vi "validate line configuration.vi"(7 "EthernetIP configuration":refnum<class "EthernetIP configuration.lvclass">, 11 "line in":T1) -> (1 "valid?":bool, 2 "problem":string, 3 "line out":T1)   [LabVIEW 2013, in "EthernetIP editor node.lvclass"]
uses:
  EthernetIP editor node.lvclass
  table line.ctl
  <vilib>/NI/TBM Modules/Ethernet IP/channel/EthernetIP Channel.lvclass
  <vilib>/NI/TBM Modules/Ethernet IP/configuration/EthernetIP configuration.lvclass
  <vilib>/NI/Tag Bus/tag/tag descriptor.lvclass/tag descriptor.ctl
  <vilib>/NI/TBM Modules/Ethernet IP/channel/EthernetIP Channel.lvclass/EthernetIP Channel.ctl
  <vilib>/NI/Tag Bus Module Framework/channel/TBM channel.lvclass/TBM channel.ctl
  <vilib>/NI/TBM Modules/Ethernet IP/configuration/EthernetIP configuration.lvclass/EthernetIP configuration.ctl
  <vilib>/NI/TBM Modules/Ethernet IP/configuration/read eip channels.vi
  <vilib>/NI/TBM Modules/Ethernet IP/configuration/Read assemblies.vi
  <vilib>/NI/Tag Bus/tag/read tag name.vi
  <vilib>/NI/TBM Modules/Ethernet IP/channel/Read Instance ID.vi
  <vilib>/NI/Tag Bus Module Framework/channel/Read channel classification.vi
  <vilib>/NI/TBM Modules/Ethernet IP/channel/Read subindex.vi
  <vilib>/NI/Tag Bus/tag/tag descriptor.lvclass
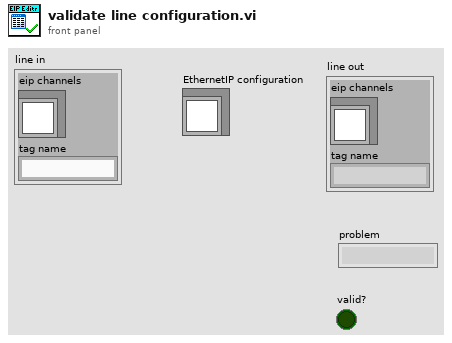
[diagram p1: front panel]
types:
  T1 = typedef "EthernetIP editor node.lvclass/table line.ctl" = cluster{"eip channels":refnum<class "EthernetIP Channel.lvclass">, "tag name":string}
  T2 = typedef "TBM channel.lvclass/channel classification.ctl" = enum16{"input data", "output data", "processing parameter", "processing result"}
  T3 = typedef "EthernetIP configuration.lvclass/assembly definition.ctl" = cluster{"name":string, "Instance ID":u32, "Type":T4, "Size (bytes)":u32}
  T4 = typedef "EthernetIP configuration.lvclass/assembly type.ctl" = enum32{"Producing", "Consuming"}
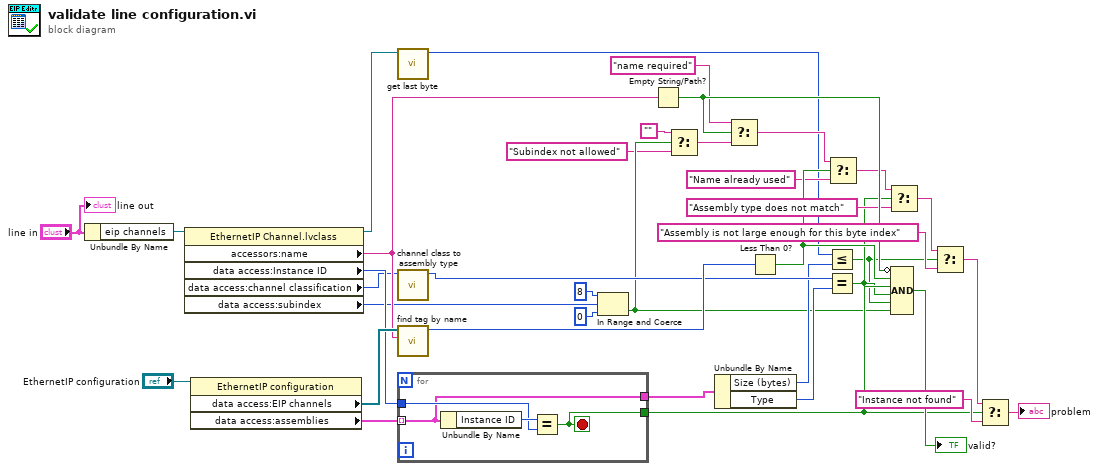
[diagram p0: block diagram]
diagram:
  n1 = Unbundle By Name("line in") -> ("eip channels"=w37:refnum<class "EthernetIP Channel.lvclass">)
  n2 = property class="EthernetIP Channel.lvclass"(reference=w37) -> (reference out=w11:refnum<class "EthernetIP Channel.lvclass">, "accessors:name"=w34:string, "data access:Instance ID"=w25:u32, "data access:channel classification"=w22:T2, "data access:subindex"=w7:i32)  [unwired: 1 in, 1 out]
  n3 = property class="EthernetIP configuration"(reference="EthernetIP configuration") -> ("data access:EIP channels"=w35:refnum<class "EthernetIP Channel.lvclass">[], "data access:assemblies"=w31:T3[])  [unwired: 1 in, 2 out]
  n4 = call <vilib>:"get last byte.vi"("EthernetIP Channel in"=w11) -> ("last byte"=w10:i32)  [unwired: 10 in]
  n5 = call <vilib>:"channel class to assembly type.vi"("channel classification"=w22) -> ("assembly types"=w13:T4)  [unwired: 10 in]
  n6 = call <vilib>:"find tag by name.vi"("name"=w34, "tags in"=w35) -> ("index"=w32:i32)  [unwired: 9 in]
  n7 = for {
    tunnel: w31 -> [w40] mode=indexing
    tunnel: w25 -> [w41]
    tunnel: [w40] -> w18
    tunnel: [w39] -> w23
    stop <- w39 stop-if-true
    n8 = Unbundle By Name(w40) -> ("Instance ID"=w42:u32)
    n9 = Equal?(x=w42, y=w41) -> (x = y?=w39:bool)
  }
  n10 = In Range and Coerce(upper limit=8, x=w7, lower limit=0) -> (In Range?=w2:bool)  [unwired: 1 out]
  n11 = Empty String/Path?(string/path=w34) -> (empty?=w30:bool)
  n12 = Select(t="", s=w2, f="Subindex not allowed") -> (s? t:f=w3:string)
  n13 = Unbundle By Name(w18) -> ("Size (bytes)"=w9:u32, "Type"=w14:T4)
  n14 = Select(t="name required", s=w30, f=w3) -> (s? t:f=w28:string)
  n15 = Less Than 0?(x=w32) -> (x < 0?=w29:bool)
  n16 = Less Or Equal?(x=w10, y=w9) -> (x <= y?=w8:bool)
  n17 = Equal?(x=w13, y=w14) -> (x = y?=w12:bool)
  n18 = Select(t=w28, s=w29, f="Name already used") -> (s? t:f=w17:string)
  n19 = Select(t=w17, s=w12, f="Assembly type does not match") -> (s? t:f=w19:string)
  n20 = Compound Arithmetic op=AND(invert w30, w29, w23, w12, w8, w2) -> (→"valid?":bool)
  n21 = Select(t=w19, s=w8, f="Assembly is not large enough for this byte index") -> (s? t:f=w16:string)
  n22 = Select(t=w16, s=w23, f="Instance not found") -> (s? t:f=→"problem":string)
  "line out" <- "line in"
